vi "get encoder pos.vi"(8 "error in (no error)":errorcluster, 11 "ch":i32) -> (0 "error out":errorcluster, 3 "Output Angle":dbl)   [LabVIEW 2014, in "test_IMU.lvlib"]
doc: "int get_encoder_pos(int ch);"
uses:
  <userlib>/test_IMU/test_IMU.lvlib
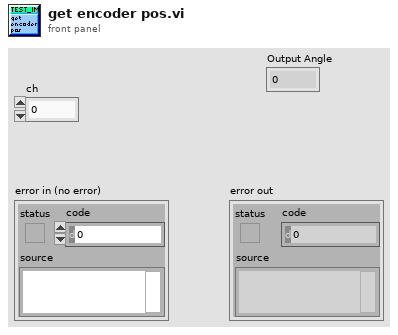
[diagram p1: front panel]
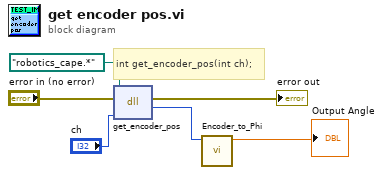
[diagram p0: block diagram]
diagram:
  # "int get_encoder_pos(int ch);"
  n1 = dll-call lib="C:/Users/ktalke/Documents/Updated Header File/6.18.16/Compiled SO -schroot/robotics_cape.so" fn="get_encoder_pos"(path in=path "robotics_cape.*", error in="error in (no error)", "ch"="ch") -> (error out=→"error out":errorcluster, "return type"=w2:i32)  [unwired: 2 in, 1 out]
  n2 = call <userlib>:"Encoder_to_Phi.vi"("Encoder Output"=w2) -> ("Output Angle"=→"Output Angle":dbl)  [unwired: 10 in]
